vi "GlobalDAQconnected.vi"() -> ()   [LabVIEW 2022 SP3]
panel:
  in  "Boolean":bool
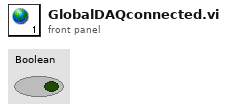
[diagram p1: front panel]
diagram:
